vi "UserInterfaceInvertedPendulum.vi"() -> ()   [LabVIEW 2009]
uses:
  <vilib>/picture/picture.llb/Draw True-Color Pixmap.vi
  <vilib>/Utility/file.llb/Write To Spreadsheet File (DBL).vi
  <vilib>/Utility/file.llb/Write To Spreadsheet File (string).vi
panel:
  out "KTH  Automatic Control \nWireless Process Control over IEEE 802.15.4":picture
  in  "Tab Control":T1(tab)
  out "reliability =pckSuccess/pckTotal":dynamicdata(graph)
  out "errors":dynamicdata(graph)
  out "Inter sampling time = t_k - t_k-1":dynamicdata(graph)
  out "delay = t_send - t_ack":dynamicdata(graph)
  out "x":dynamicdata(graph)
  out "Control output":dynamicdata(graph)
  out "Theta angle":dynamicdata(graph)
  in  "StartSaving":bool
  in  "Saving":bool
  in  "StopSaving":bool
  out "Path":path
  out "xc_value":dbl
  out "theta_value":dbl
  out "errors_u":dbl
  out "errors_theta":dbl
  out "delay_xc":dbl
  out "delay_u":dbl
  out "delay_theta":dbl
  out "interSampling_xc":dbl
  out "interSampling_theta":dbl
  out "interSampling_u":dbl
  out "errors_xc":dbl
  out "reliability_u":dbl
  out "reliability_xc":dbl
  out "reliability_theta":dbl
  out "control_output":dbl
  out "current time":timestamp
  out "Packet Window":i32=200
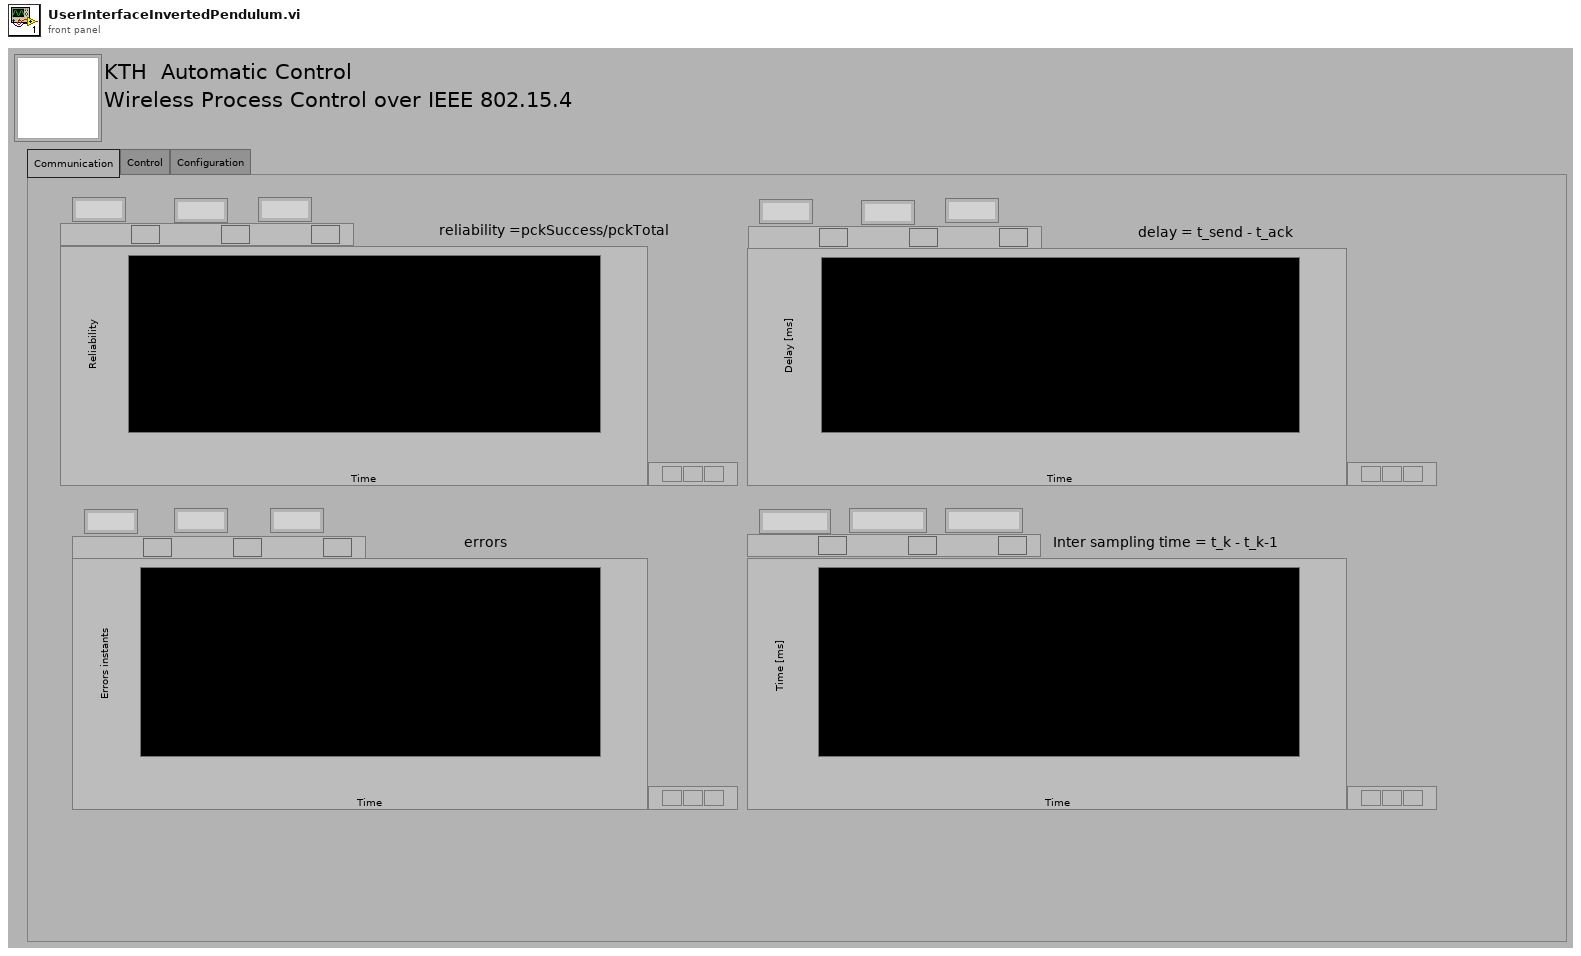
[diagram p1: front panel]
types:
  T1 = enum32{"Communication", "Control", "Configuration"}
  T2 = enum8{"Enabled", "Disabled", "Disabled and Grayed Out"}
  T3 = typedef "imagedata.ctl" = cluster{"image type":i32, "image depth":i32, "image":u8[], "mask":u8[], "colors":u32[], "Rectangle":cluster{"left":i16, "top":i16, "right":i16, "bottom":i16}}
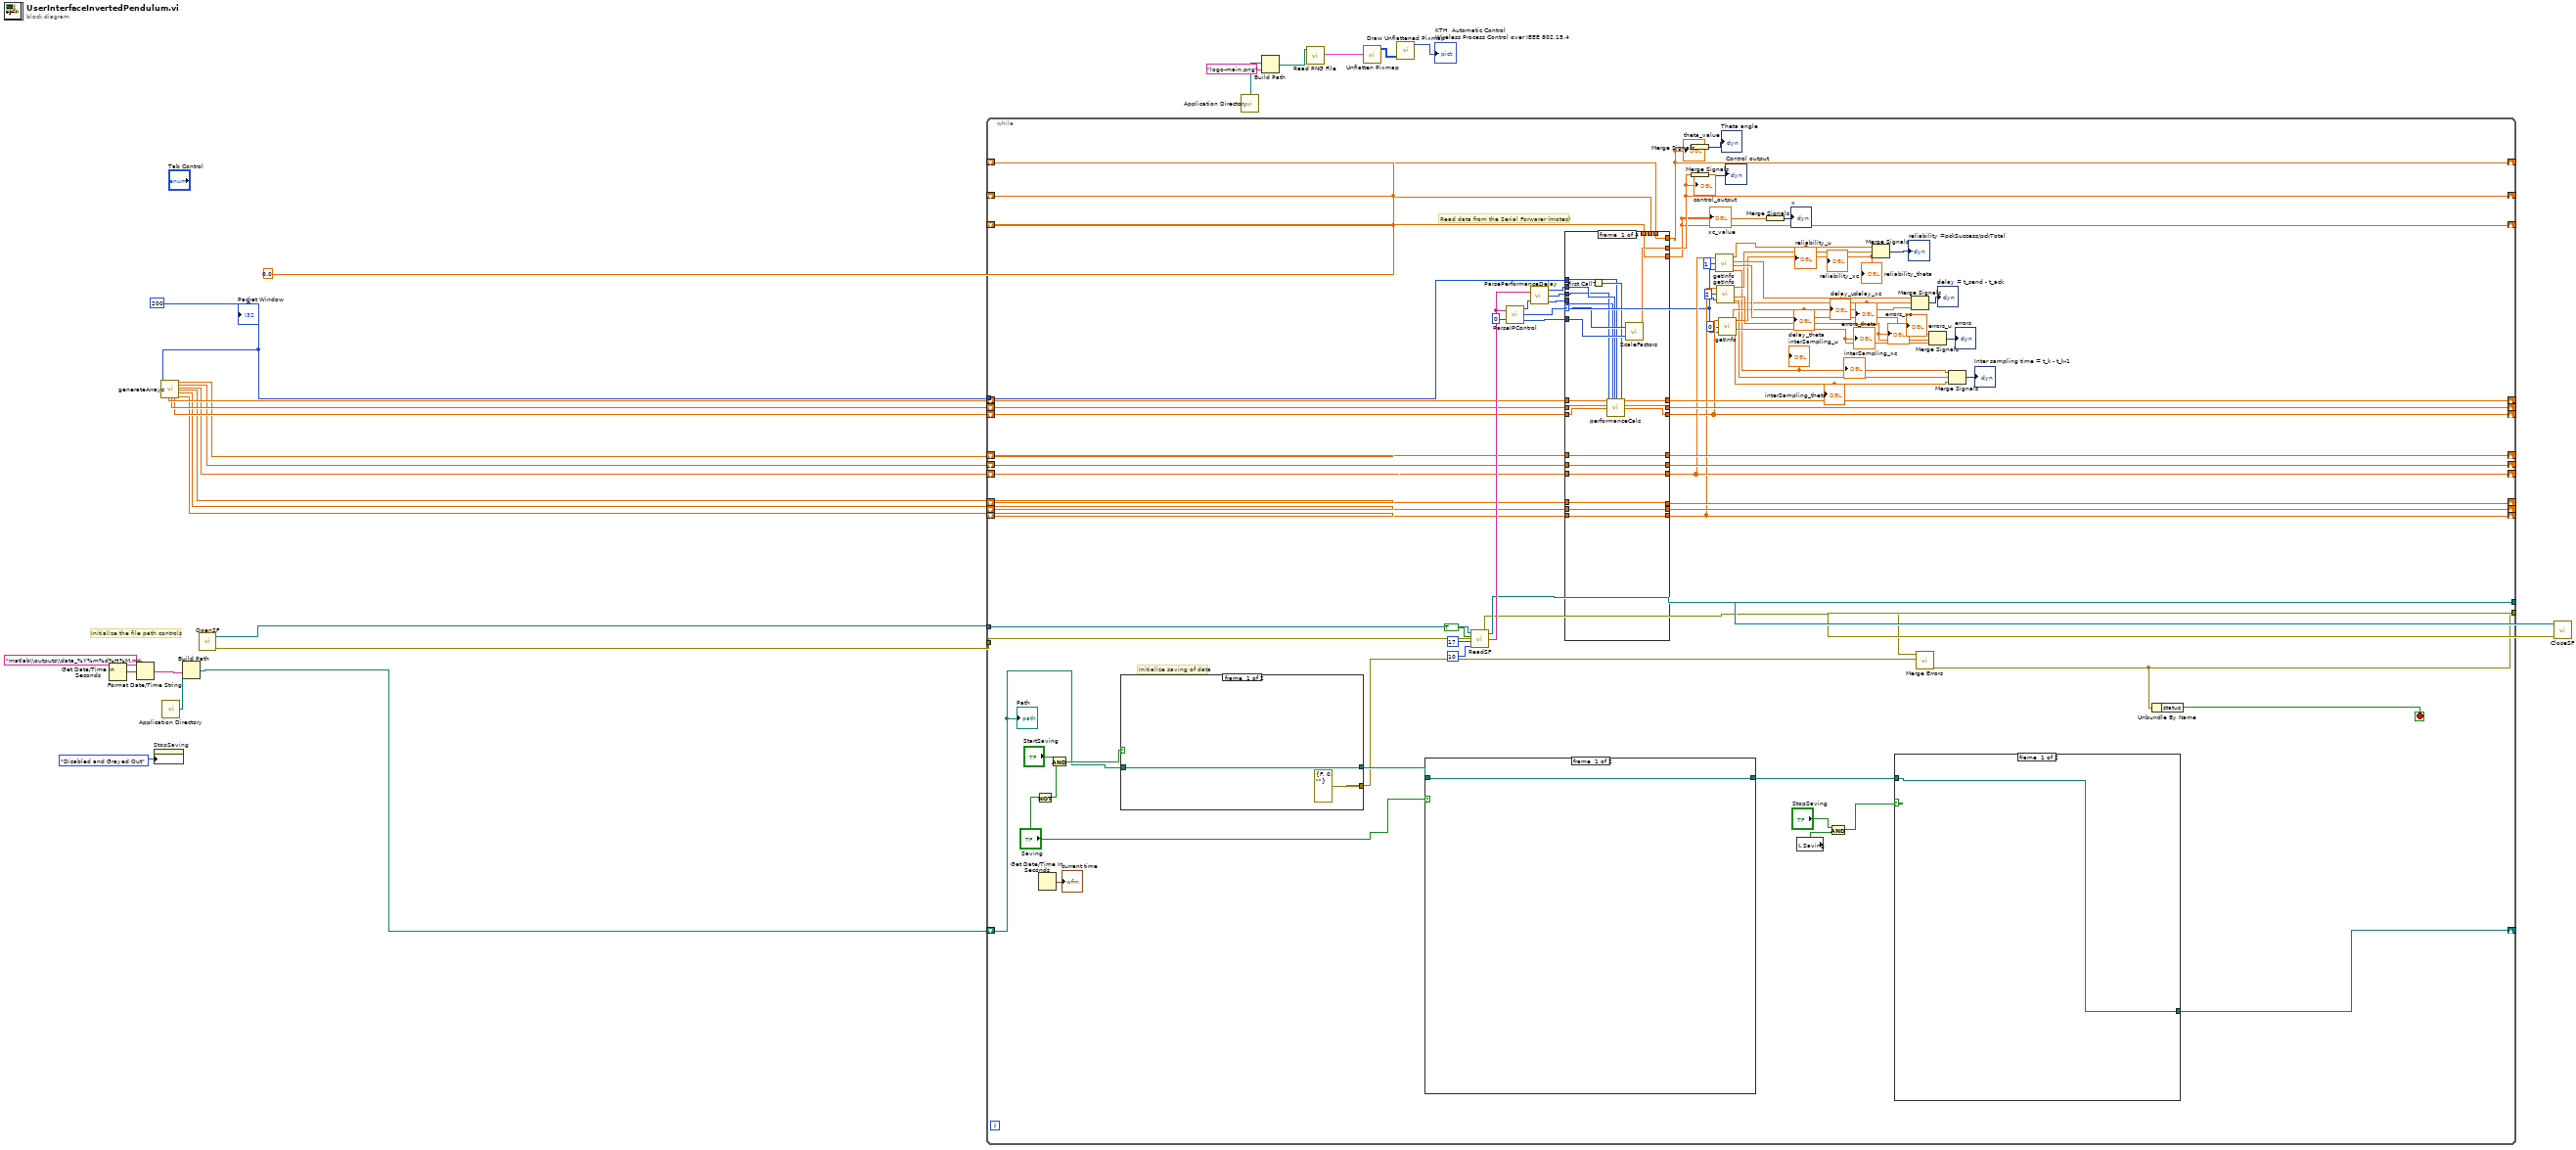
[diagram p0: block diagram]
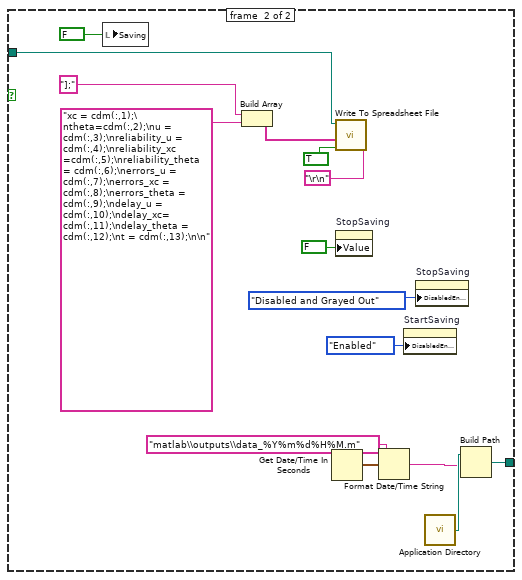
[diagram p2: hidden frame]
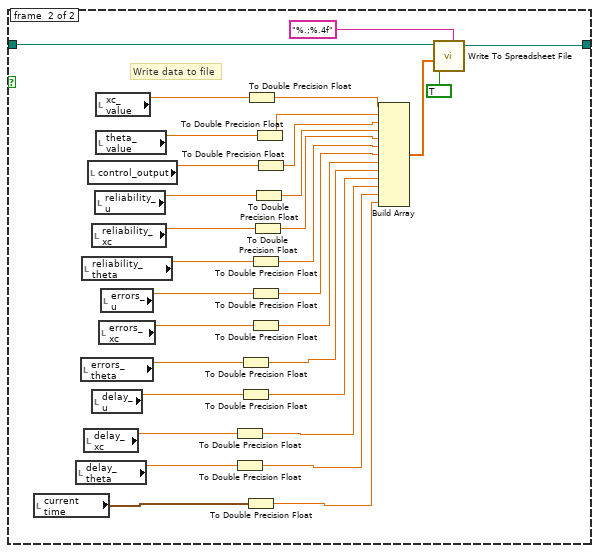
[diagram p3: hidden frame]
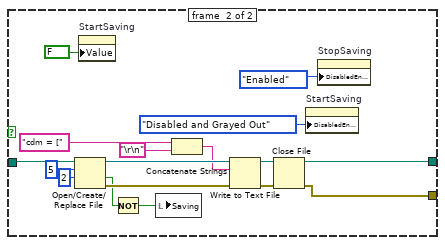
[diagram p4: hidden frame]
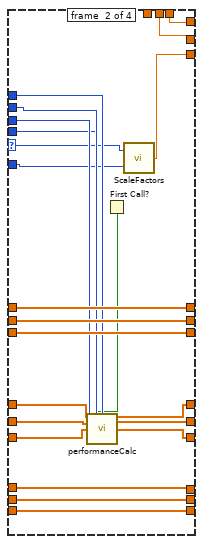
[diagram p5: hidden frame]
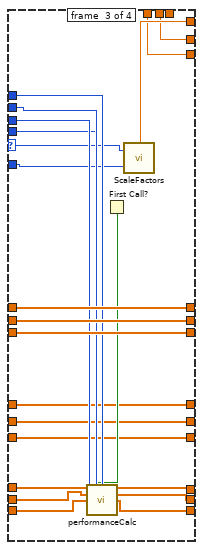
[diagram p6: hidden frame]
diagram:
  w24 = 200 ("Packet Window")
  w14 = 0.0 ("prevPckTotalOut")
  # "Initialize the file path controls"
  n1 = Get Date/Time In Seconds() -> (seconds since 1Jan1904=w12:timestamp)
  n2 = Format Date/Time String(time format string (%c)="matlab\\outputs\\data_%Y%m%d%H%M.m", seconds (now)=w12) -> (date/time string=w10:string)  [unwired: 1 in]
  n3 = property on="StopSaving" class="Bool (strict)"("DisabledEnum"=T2."Disabled and Grayed Out" ("Disabled")) -> ()  [unwired: 2 in, 2 out]
  n4 = call "generateArrays.vi"("dimension size"=w24) -> ("errorsWindow1"=w23:dbl[], "pckTotalTrack1"=w22:dbl[], "state1"=w21:dbl[], "errorsWindow2"=w20:dbl[], "pckTotalTrack2"=w19:dbl[], "state2"=w18:dbl[], "errorsWindow3"=w17:dbl[], "pckTotalTrack3"=w16:dbl[], "state3"=w15:dbl[])  [unwired: 10 in]
  n5 = call <vilib>:"Application Directory.vi"() -> ("Application Directory"=w13:path)
  n6 = Build Path(base path=w13, name or relative path=w10) -> (appended path=w7:path)
  n7 = call "OpenSF.vi"() -> ("error out"=w26:errorcluster, "connection ID"=w27:refnum<k5>)  [unwired: 1 out]
  n8 = while {
    tunnel: w27 -> [w87]
    tunnel: w26 -> [w104]
    tunnel: [w86] -> w25
    tunnel: [w38] -> w9
    tunnel: w24 -> [w97]
    shift-right: [w82] -> _
    shift-left: w23 -> [w80]
    shift-right: [w81] -> _
    shift-left: w22 -> [w79]
    shift-right: [w65] -> _
    shift-left: w14 -> [w85]
    shift-right: [w66] -> _
    shift-left: w14 -> [w67]
    shift-right: [w84] -> _
    shift-left: w14 -> [w68]
    shift-right: [w54] -> _
    shift-left: w21 -> [w78]
    shift-right: [w74] -> _
    shift-left: w20 -> [w77]
    shift-right: [w73] -> _
    shift-left: w19 -> [w76]
    shift-right: [w56] -> _
    shift-left: w18 -> [w75]
    shift-right: [w69] -> _
    shift-left: w17 -> [w72]
    shift-right: [w55] -> _
    shift-left: w16 -> [w71]
    shift-right: [w53] -> _
    shift-left: w15 -> [w70]
    shift-right: [w29] -> _
    shift-left: w7 -> [w28]
    stop <- w37 stop-if-true
    # "Initialize saving of data"
    # "Read data from the Serial Forwarer (motes)"
    n9 = Not(x="Saving") -> (.not. x?=w34:bool)
    n10 = Get Date/Time In Seconds() -> (seconds since 1Jan1904=→"current time":timestamp)
    n11 = And(x="StartSaving", y=w34) -> (x .and. y?=w35:bool)
    n12 = case shown="True" w35 {
      tunnel: w28 -> [w154 w163]
      tunnel: [w154 w160] -> w44
      tunnel: [errorcluster {"status"=FALSE, "code"=0, "source"=""} ("error out") w157] -> w39
      frame #0 {
      }
      frame #1 {
        n13 = Open/Create/Replace File(file path (use dialog)=w163, operation (0:open)=5, access (0:read/write)=2) -> (refnum out=w169:refnum<file>, cancelled=w162:bool, error out=w166:errorcluster)  [unwired: 3 in]
        n14 = property on="StartSaving" class="Bool (strict)"("Value"=FALSE ("StartSaving")) -> ()  [unwired: 2 in, 2 out]
        n15 = Not(x=w162) -> (.not. x?=w159:bool)
        n16 = local write "Saving"(w159) -> ()
        n17 = Concatenate Strings("cdm = [", "\r\n") -> (w165:string)
        n18 = Write to Text File(file (use dialog)=w169, text=w165, error in=w166) -> (refnum out=w168:refnum<file>, error out=w167:errorcluster)  [unwired: 1 in, 1 out]
        n19 = Close File(refnum=w168, error in=w167) -> (path=w160:path, error out=w157:errorcluster)
        n20 = property on="StartSaving" class="Bool (strict)"("DisabledEnum"=T2."Disabled and Grayed Out" ("Disabled")) -> ()  [unwired: 2 in, 2 out]
        n21 = property on="StopSaving" class="Bool (strict)"("DisabledEnum"=T2."Enabled" ("Disabled")) -> ()  [unwired: 2 in, 2 out]
      }
    }
    n22 = case shown="True" "Saving" {
      tunnel: w44 -> [w121 w151]
      tunnel: [w121 w122] -> w41
      frame #0 {
      }
      frame #1 {
        # "Write data to file"
        n23 = local read "current time"() -> (w123:timestamp)
        n24 = local read "delay_theta"() -> (w131:dbl)
        n25 = local read "errors_theta"() -> (w132:dbl)
        n26 = local read "reliability_theta"() -> (w140:dbl)
        n27 = local read "delay_xc"() -> (w130:dbl)
        n28 = local read "control_output"() -> (w145:dbl)
        n29 = local read "reliability_xc"() -> (w141:dbl)
        n30 = local read "delay_u"() -> (w133:dbl)
        n31 = local read "reliability_u"() -> (w143:dbl)
        n32 = local read "xc_value"() -> (w149:dbl)
        n33 = local read "theta_value"() -> (w147:dbl)
        n34 = local read "errors_xc"() -> (w136:dbl)
        n35 = local read "errors_u"() -> (w139:dbl)
        n36 = To Double Precision Float(number=w130) -> (double precision float=w127:dbl)
        n37 = To Double Precision Float(number=w131) -> (double precision float=w126:dbl)
        n38 = To Double Precision Float(number=w132) -> (double precision float=w129:dbl)
        n39 = To Double Precision Float(number=w133) -> (double precision float=w128:dbl)
        n40 = To Double Precision Float(number=w123) -> (double precision float=w124:dbl)
        n41 = To Double Precision Float(number=w149) -> (double precision float=w148:dbl)
        n42 = To Double Precision Float(number=w140) -> (double precision float=w137:dbl)
        n43 = To Double Precision Float(number=w139) -> (double precision float=w135:dbl)
        n44 = To Double Precision Float(number=w136) -> (double precision float=w134:dbl)
        n45 = To Double Precision Float(number=w141) -> (double precision float=w138:dbl)
        n46 = To Double Precision Float(number=w143) -> (double precision float=w142:dbl)
        n47 = To Double Precision Float(number=w147) -> (double precision float=w146:dbl)
        n48 = To Double Precision Float(number=w145) -> (double precision float=w144:dbl)
        n49 = Build Array(w148, w146, w144, w142, w138, w137, w135, w134, w129, w128, w127, w126, w124) -> (w125:dbl[])
        n50 = call-poly <vilib>:"Write To Spreadsheet File.vi"("format (%.3f)"="%.;%.4f", "append to file? (new file:F)"=TRUE, "1D data"=w125, "file path (dialog if empty)"=w151) -> ("new file path (Not A Path if cancelled)"=w122:path)  [unwired: 4 in]
      }
    }
    n51 = call "ReadSF.vi"("connection ID in"=w87, "enabled"=TRUE, "bytes to read"=17 ("f"), "header size"=10 ("bytes to read"), "error in"=w104) -> ("connection ID out"=w86:refnum<k5>, "string"=w99:string, "error out"=w40:errorcluster)
    n52 = call "ParseIPControl.vi"("data out"=w99, "offset"=u8 0) -> ("Bytes Read"=w100:i32, "srcId"=w49:u8, "data"=w92:i16)
    n53 = call "ParsePerformanceDelay.vi"("data out"=w99, "offset"=w100) -> ("pckTotal"=w95:u16, "pckSuccess"=w96:u16, "delay"=w88:u16)
    n54 = case shown="0" w49 {
      selector: w49 -> [w193 w198 w229 _]
      tunnel: w92 -> [w192 w197 w228 _]
      tunnel: [w191 w195 w226 w239] -> w84
      tunnel: w97 -> [w189 w206 w234 _]
      tunnel: w96 -> [w187 w205 w233 _]
      tunnel: w95 -> [w188 w204 w232 _]
      tunnel: w88 -> [w186 w203 w231 _]
      tunnel: w85 -> [w172 _ w225 w238]
      tunnel: w68 -> [_ w195 w226 w239]
      tunnel: w67 -> [w173 w196 _ w240]
      tunnel: [w182 w215 w237 w249] -> w82
      tunnel: [w181 w214 w236 w248] -> w81
      tunnel: [w180 w213 w235 w247] -> w54
      tunnel: w80 -> [w185 w215 w237 w249]
      tunnel: w79 -> [w184 w214 w236 w248]
      tunnel: w78 -> [w183 w213 w235 w247]
      tunnel: w77 -> [w179 w209 w218 w246]
      tunnel: w76 -> [w178 w208 w217 w245]
      tunnel: w75 -> [w177 w207 w216 w244]
      tunnel: [w179 w202 w218 w246] -> w74
      tunnel: [w178 w201 w217 w245] -> w73
      tunnel: [w177 w200 w216 w244] -> w56
      tunnel: w72 -> [w176 w212 w224 w243]
      tunnel: w71 -> [w175 w211 w223 w242]
      tunnel: w70 -> [w174 w210 w222 w241]
      tunnel: [w176 w212 w221 w243] -> w69
      tunnel: [w175 w211 w220 w242] -> w55
      tunnel: [w174 w210 w219 w241] -> w53
      tunnel: [w173 w196 w227 w240] -> w66
      tunnel: [w172 w194 w225 w238] -> w65
      frame #0 {
        n55 = First Call?() -> (First Call?: T/F=w190:bool)
        n56 = call "performanceCalc.vi"("errors"=w185, "init"=w190, "windowLength"=w189, "pckTotalTrack"=w184, "state"=w183, "pckSuccess"=w187, "pckTotal"=w188, "delay"=w186) -> ("errorsOut"=w182:dbl[], "pckTotalTrackOut"=w181:dbl[], "prevState"=w180:dbl[])  [unwired: 5 in]
        n57 = call "ScaleFactors.vi"("data"=w192, "srcId"=w193) -> ("dataOut"=w191:dbl)
      }
      frame #1 {
        n58 = First Call?() -> (First Call?: T/F=w199:bool)
        n59 = call "performanceCalc.vi"("errors"=w209, "init"=w199, "windowLength"=w206, "pckTotalTrack"=w208, "state"=w207, "pckSuccess"=w205, "pckTotal"=w204, "delay"=w203) -> ("errorsOut"=w202:dbl[], "pckTotalTrackOut"=w201:dbl[], "prevState"=w200:dbl[])  [unwired: 5 in]
        n60 = call "ScaleFactors.vi"("data"=w197, "srcId"=w198) -> ("dataOut"=w194:dbl)
      }
      frame #2 {
        n61 = First Call?() -> (First Call?: T/F=w230:bool)
        n62 = call "performanceCalc.vi"("errors"=w224, "init"=w230, "windowLength"=w234, "pckTotalTrack"=w223, "state"=w222, "pckSuccess"=w233, "pckTotal"=w232, "delay"=w231) -> ("errorsOut"=w221:dbl[], "pckTotalTrackOut"=w220:dbl[], "prevState"=w219:dbl[])  [unwired: 5 in]
        n63 = call "ScaleFactors.vi"("data"=w228, "srcId"=w229) -> ("dataOut"=w227:dbl)
      }
      frame #3 {
      }
    }
    "xc_value" <- w65
    "control_output" <- w84
    "theta_value" <- w66
    n64 = Merge Signals(w66) -> (→"Theta angle":dynamicdata)
    n65 = Merge Signals(w84) -> (→"Control output":dynamicdata)
    n66 = call "getInfo.vi"("array"=w56, "srcID"=u16 1, "srcIDPck"=w49) -> ("reliability"=w64:dbl, "delay"=w63:dbl, "errors"=w62:dbl, "interSampling"=w47:dbl)
    "reliability_u" <- w64
    "errors_u" <- w62
    "interSampling_u" <- w47
    "delay_u" <- w63
    n67 = call "getInfo.vi"("array"=w53, "srcID"=u16 2, "srcIDPck"=w49) -> ("reliability"=w61:dbl, "delay"=w43:dbl, "errors"=w60:dbl, "interSampling"=w46:dbl)
    "reliability_xc" <- w61
    "errors_xc" <- w60
    "interSampling_xc" <- w46
    "delay_xc" <- w43
    n68 = call "getInfo.vi"("array"=w54, "srcID"=u16 0, "srcIDPck"=w49) -> ("reliability"=w59:dbl, "delay"=w58:dbl, "errors"=w57:dbl, "interSampling"=w45:dbl)
    "reliability_theta" <- w59
    "errors_theta" <- w57
    "interSampling_theta" <- w45
    "delay_theta" <- w58
    n69 = Merge Signals(w65) -> (→"x":dynamicdata)
    n70 = local read "Saving"() -> (w30:bool)
    n71 = And(x="StopSaving", y=w30) -> (x .and. y?=w31:bool)
    n72 = Merge Signals(w64, w61, w59) -> (→"reliability =pckSuccess/pckTotal":dynamicdata)
    n73 = case shown="True" w31 {
      tunnel: w41 -> [w105 w113]
      tunnel: [w105 w106] -> w29
      frame #0 {
      }
      frame #1 {
        n74 = local write "Saving"(FALSE) -> ()
        n75 = Build Array("];", "xc = cdm(:,1);\ntheta=cdm(:,2);\nu = cdm(:,3);\nreliability_u = cdm(:,4);\nreliability_xc =cdm(:,5);\nreliability_theta  = cdm(:,6);\nerrors_u = cdm(:,7);\nerrors_xc = cdm(:,8);\nerrors_theta = cdm(:,9);\ndelay_u = cdm(:,10);\ndelay_xc= cdm(:,11);\ndelay_theta = cdm(:,12);\nt = cdm(:,13);\n\n") -> (w118:string[])
        n76 = Get Date/Time In Seconds() -> (seconds since 1Jan1904=w109:timestamp)
        n77 = call-poly <vilib>:"Write To Spreadsheet File.vi"("delimiter (\\t)"="\r\n", "append to file? (new file:F)"=TRUE, "1D data"=w118, "file path (dialog if empty)"=w113) -> ()  [unwired: 4 in, 1 out]
        n78 = property on="StopSaving" class="Bool (strict)"("Value"=FALSE ("StartSaving")) -> ()  [unwired: 2 in, 2 out]
        n79 = Format Date/Time String(time format string (%c)="matlab\\outputs\\data_%Y%m%d%H%M.m", seconds (now)=w109) -> (date/time string=w107:string)  [unwired: 1 in]
        n80 = property on="StartSaving" class="Bool (strict)"("DisabledEnum"=T2."Enabled" ("Disabled")) -> ()  [unwired: 2 in, 2 out]
        n81 = property on="StopSaving" class="Bool (strict)"("DisabledEnum"=T2."Disabled and Grayed Out" ("Disabled")) -> ()  [unwired: 2 in, 2 out]
        n82 = call <vilib>:"Application Directory.vi"() -> ("Application Directory"=w110:path)
        n83 = Build Path(base path=w110, name or relative path=w107) -> (appended path=w106:path)
      }
    }
    n84 = Merge Signals(w63, w43, w58) -> (→"delay = t_send - t_ack":dynamicdata)
    n85 = call <vilib>:"Merge Errors.vi"("error in 2 (no error)"=w39, "error in 1 (no error)"=w40) -> ("error out"=w38:errorcluster)  [unwired: 5 in]
    n86 = Merge Signals(w62, w60, w57) -> (→"errors":dynamicdata)
    n87 = Merge Signals(w47, w46, w45) -> (→"Inter sampling time = t_k - t_k-1":dynamicdata)
    n88 = Unbundle By Name(w38) -> ("status"=w37:bool)
    "Path" <- w28
  }
  n89 = call <vilib>:"Application Directory.vi"() -> ("Application Directory"=w2:path)
  n90 = Build Path(base path=w2, name or relative path="logo-main.png") -> (appended path=w3:path)
  n91 = call <vilib>:"Read PNG File.vi"("path to PNG file"=w3) -> ("image data"=w6:T3)  [unwired: 8 in, 2 out]
  n92 = call <vilib>:"Unflatten Pixmap.vi"("image data"=w6) -> ("24-bit pixmap"=w5:u32[][])  [unwired: 4 in, 6 out]
  n93 = call-poly <vilib>:"Draw Unflattened Pixmap.vi"("data (RGB format)"=w5) -> ("new picture"=→"KTH  Automatic Control \nWireless Process Control over IEEE 802.15.4":picture)  [unwired: 8 in]
  n94 = call "CloseSF.vi"("error out"=w9, "connection ID"=w25) -> ()  [unwired: 1 in]
  "Packet Window" <- w24
